vi "OP500ZP_BDD.vi"(8 "errin":errorcluster, 10 "DATA IN":T1) -> (0 "error out":errorcluster)   [LabVIEW 2020]
panel:
  out "chaîne concaténée":string
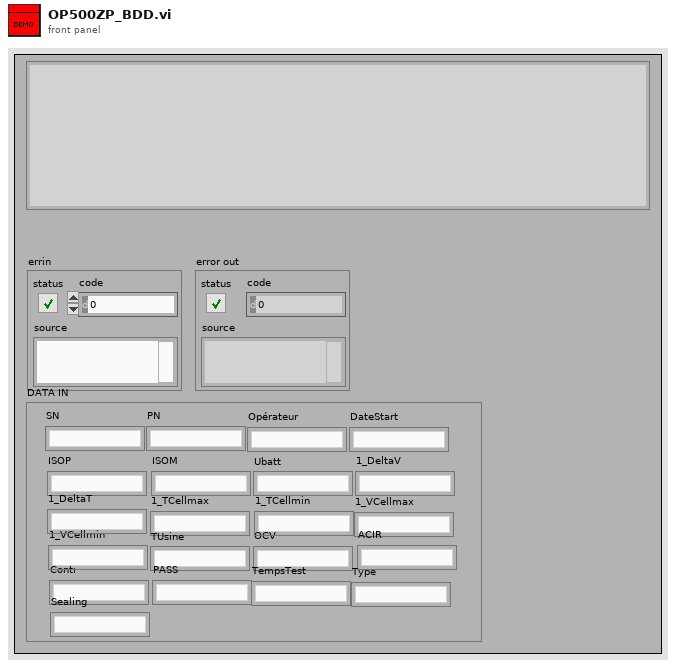
[diagram p1: front panel]
types:
  T1 = cluster{"SN":string, "PN":string, "Opérateur":string, "DateStart":string, "ISOP":string, "ISOM":string, "Ubatt":string, "1_DeltaV":string, "1_DeltaT":string, "1_TCellmax":string, "1_TCellmin":string, "1_VCellmax":string, "1_VCellmin":string, "TUsine":string, "OCV":string, "ACIR":string, "Conti":string, "PASS":string, "TempsTest":string, "Type":string, "Sealing":string}
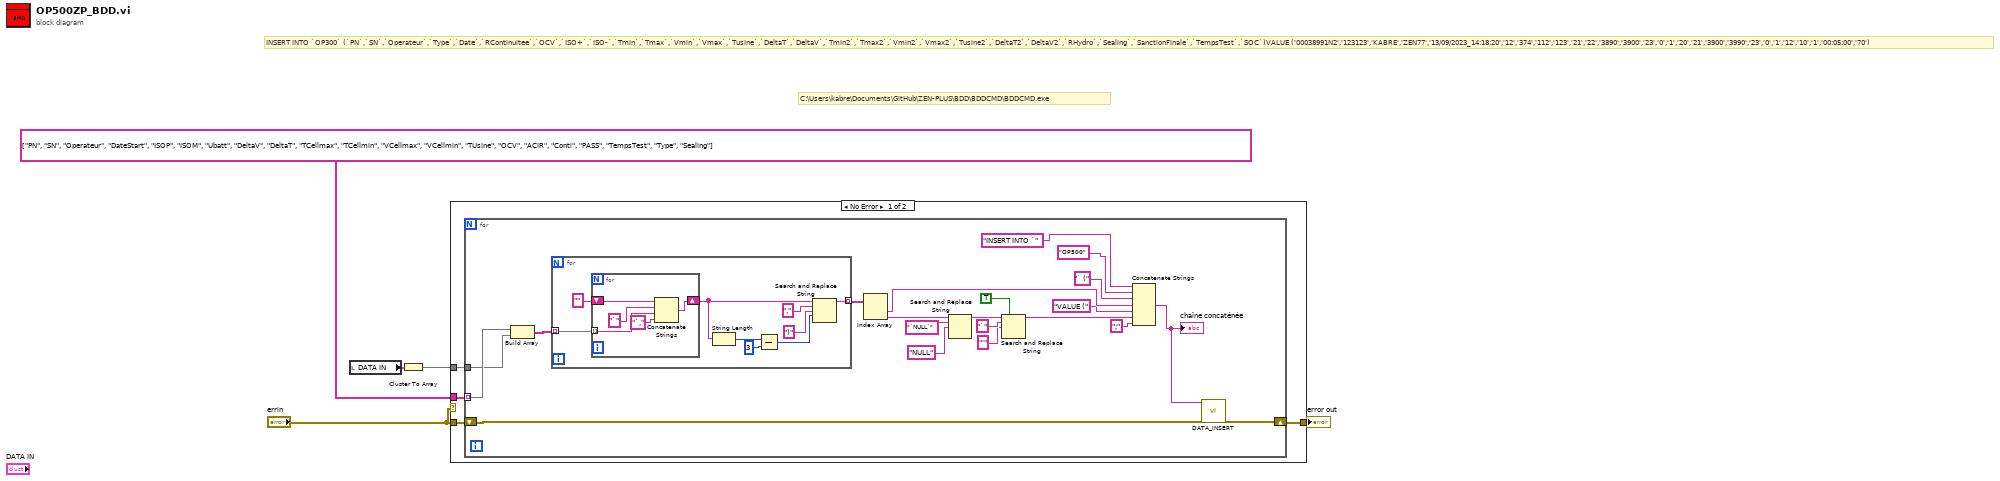
[diagram p0: block diagram]
diagram:
  # "INSERT INTO `OP300` (`PN`,`SN`,`Operateur`,`Type`,`Date`,`RContinuitee`,`OCV`,`ISO+`,`ISO-`,`Tmin`,`Tmax`,`Vmin`,`Vmax`,`Tusine`,`DeltaT`,`DeltaV`,`Tmin2`,`Tmax2`,`Vmin2`,`Vmax2`,`Tusine2`,`DeltaT2`,`DeltaV2`,`RHydro`,`Sealing`,`SanctionFinale`,`TempsTest`,`SOC`)VALUE ('00038991N2','123123','KABRE','ZEN77','13/09/2023_14:18:20','12','374','112','123','21','22','3890','3900','23','0','1','20','21','3900','3990','23','0','1','12','10','1','00:05:00','70')"
  # "C:\\Users\\kabre\\Documents\\GitHub\\ZEN-PLUS\\BDD\\BDDCMD\\BDDCMD.exe"
  n1 = local read "DATA IN"() -> (w1:T1)
  n2 = Cluster To Array(cluster=w1) -> (array=w2:string[])
  n3 = case shown="No Error" "errin" {
    tunnel: "errin" -> [w9 w45]
    tunnel: [w8 w45] -> w5
    tunnel: string[][] [["PN", "SN", "Operateur", "DateStart", "ISOP", "ISOM", "Ubatt", "DeltaV", "DeltaT", "TCellmax", "TCellmin", "VCellmax", "VCellmin", "TUsine", "OCV", "ACIR", "Conti", "PASS", "TempsTest", "Type", "Sealing"]] -> [w7 _]
    tunnel: w2 -> [w6 _]
    frame No Error {
      n4 = for {
        shift-right: [w11] -> w8
        shift-left: w9 -> [w12]
        tunnel: w7 -> [w15] mode=indexing
        tunnel: w6 -> [w14]
        n5 = Build Array(w15, w14) -> (w30:string[][])
        n6 = for {
          tunnel: [w31] -> w16 mode=indexing
          tunnel: w30 -> [w39] mode=indexing
          n7 = for {
            shift-right: [w42] -> w32
            shift-left: "" -> [w41]
            tunnel: w39 -> [w40] mode=indexing
            n8 = Concatenate Strings(w41, "`" ("string"), w40, "`," ("string")) -> (w42:string)
          }
          n9 = String Length(string=w32) -> (length=w37:i32)
          n10 = Subtract(x=w37, y=3) -> (x-y=w35:i32)
          n11 = Search and Replace String(input string=w32, search string=",", replace string=")" ("replace string (\"\")"), offset=w35) -> (result string=w31:string)  [unwired: 4 in, 3 out]
        }
        n12 = Index Array(array=w16) -> (element #1=w26:string, element #2=w27:string)  [unwired: 2 in]
        n13 = Search and Replace String(input string=w27, search string="`NULL`", replace string="NULL" ("replace string (\"\")")) -> (result string=w28:string)  [unwired: 5 in, 3 out]
        n14 = Search and Replace String(replace all?=TRUE ("replace all? (F)"), input string=w28, search string="`", replace string="'" ("replace string (\"\")")) -> (result string=w29:string)  [unwired: 4 in, 3 out]
        n15 = Concatenate Strings("INSERT INTO `" ("string"), "OP500", "` (" ("string"), w26, "VALUE (" ("string"), w29, ";" ("string")) -> (w10:string)
        "chaîne concaténée" <- w10
        n16 = call <userlib>:"DATA_INSERT.vi"("errin"=w12, "INSERT"=w10) -> ("errout"=w11:errorcluster)  [unwired: 9 in]
      }
    }
    frame Error {
    }
  }
  "error out" <- w5
